vi "Open_Data_File.vi"(8 "error in (no error)":errorcluster, 11 "Number of Iterations":i32) -> (0 "error out":errorcluster, 2 "Encoder Counts":dbl, 3 "Time":dbl)   [LabVIEW 2018]
doc: "This VI reads and outputs data from a csv file which contains time values and the corresponding encoder counts.\n\nInputs:\nNo. of Iteration;\nError In.\n\nOutputs:\nError Out;\nEncoder Counts;\nTime."
uses:
  <vilib>/Utility/file.llb/Read Delimited Spreadsheet (DBL).vi
panel:
  in  "File Path":path
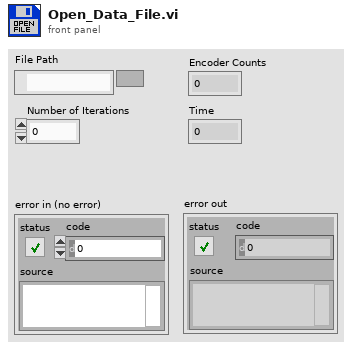
[diagram p1: front panel]
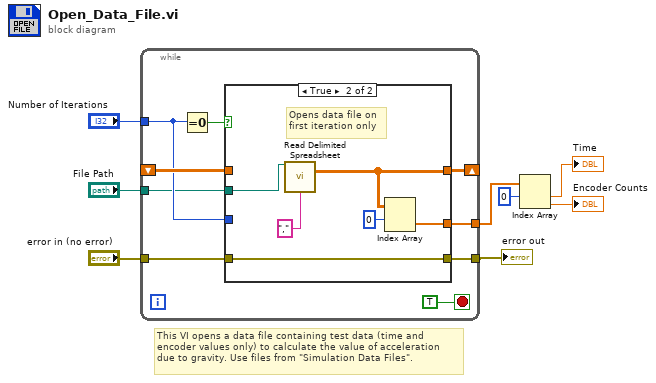
[diagram p0: block diagram]
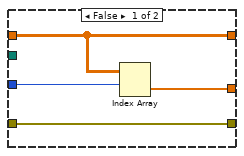
[diagram p2: hidden frame]
diagram:
  # "This VI opens a data file containing test data (time and\nencoder values only) to calculate the value of acceleration\ndue to gravity. Use files from \"Simulation Data Files\"."
  n1 = while {
    tunnel: "error in (no error)" -> [w17]
    tunnel: [w16] -> w7
    shift-right: [w14] -> _
    shift-left: _ -> [w12]
    tunnel: [w13] -> w6
    tunnel: "Number of Iterations" -> [w10]
    tunnel: "File Path" -> [w9]
    stop <- TRUE stop-if-true
    n2 = Equal To 0?(x=w10) -> (x = 0?=w11:bool)
    n3 = case shown="True" w11 {
      tunnel: w17 -> [w21 w26]
      tunnel: [w21 w26] -> w16
      tunnel: [w20 w24] -> w14
      tunnel: w12 -> [w20 _]
      tunnel: [w19 w23] -> w13
      tunnel: w10 -> [w18 _]
      tunnel: w9 -> [_ w22]
      frame False {
        n4 = Index Array(array=w20, index (row)=w18) -> (element=w19:dbl[])  [unwired: 1 in]
      }
      frame True {
        # "Opens data file on\nfirst iteration only"
        n5 = call-poly <vilib>:"Read Delimited Spreadsheet.vi"("file path (dialog if empty)"=w22, "delimiter (\\t)"="," ("delimiter (\\t)")) -> ("all rows"=w24:dbl[][])  [unwired: 8 in, 5 out]
        n6 = Index Array(array=w24, index (row)=0 ("index")) -> (element=w23:dbl[])  [unwired: 1 in]
      }
    }
  }
  "error out" <- w7
  n7 = Index Array(array=w6, index #1=0 ("index")) -> (element #1=→"Time":dbl, element #2=→"Encoder Counts":dbl)  [unwired: 1 in]
